vi "CheckForBadVIs.vi"() -> ()   [LabVIEW 2020]
panel:
  out "Bad":path[](array[path])=[path "ClassProviders/DesignPatterns/ActiveObjects/ActiveObjects_DynamicEvents_SubVIs/ActiveObjects_DynamicEvents_ControlWindow_4x4x4.vi", path "ClassProviders/DesignPatterns/ActiveObjects/ActiveObjects_DynamicEvents_SubVIs/ActiveObjects_DynamicEvents_ControlWindow_4x4x4_Singleton.vi", path "ClassProviders/DesignPatterns/ActiveObjects/ActiveObjects_DynamicEvents_SubVIs/ActiveObjects_DynamicEvents_ControlWindow_6x8x6.vi", path "ClassProviders/DesignPatterns/ActiveObjects/ActiveObjects_DynamicEvents_SubVIs/ActiveObjects_DynamicEvents_ControlWindow_6x8x6_Singleton.vi", path "ClassProviders/DesignPatterns/ActiveObjects/ActiveObjects_DynamicEvents_SubVIs/ActiveObjects_DynamicEvents_Process.vi", path "ClassProviders/DesignPatterns/ActiveObjects/ActiveObjects_DynamicEvents_SubVIs/ActiveObjects_DynamicEvents_ProcessRepository_EndevoGoop3.vi", path "ClassProviders/DesignPatterns/ActiveObjects/ActiveObjects_DynamicEvents_SubVIs/ActiveObjects_DynamicEvents_ProcessRepository_Native.vi", path "ClassProviders/DesignPatterns/ActiveObjects/ActiveObjects_DynamicEvents_SubVIs/ActiveObjects_DynamicEvents_SendMsgToProcess_4x4x4.vi", path "ClassProviders/DesignPatterns/ActiveObjects/ActiveObjects_DynamicEvents_SubVIs/ActiveObjects_DynamicEvents_SendMsgToProcess_4x4x4_Singleton.vi", path "ClassProviders/DesignPatterns/ActiveObjects/ActiveObjects_DynamicEvents_SubVIs/ActiveObjects_DynamicEvents_SendMsgToProcess_6x8x6.vi", path "ClassProviders/DesignPatterns/ActiveObjects/ActiveObjects_DynamicEvents_SubVIs/ActiveObjects_DynamicEvents_SendMsgToProcess_6x8x6_Singleton.vi", path "ClassProviders/DesignPatterns/ActiveObjects/ActiveObjects_DynamicEvents_SubVIs/ActiveObjects_DynamicEvents_StartProcess_OnePerClass.vi", path "ClassProviders/DesignPatterns/ActiveObjects/ActiveObjects_DynamicEvents_SubVIs/ActiveObjects_DynamicEvents_StartProcess_OnePerObject.vi", path "ClassProviders/DesignPatterns/ActiveObjects/ActiveObjects_DynamicEvents_SubVIs/ActiveObjects_DynamicEvents_StopProcess.vi", path "ClassProviders/DesignPatterns/ActiveObjects/ActiveObjects_Finisar_SubVIs/ActiveObjects_Finisar_ControlWindow_4x4x4.vi", path "ClassProviders/DesignPatterns/ActiveObjects/ActiveObjects_Finisar_SubVIs/ActiveObjects_Finisar_ControlWindow_4x4x4_Singleton.vi", path "ClassProviders/DesignPatterns/ActiveObjects/ActiveObjects_Finisar_SubVIs/ActiveObjects_Finisar_ControlWindow_6x8x6.vi", path "ClassProviders/DesignPatterns/ActiveObjects/ActiveObjects_Finisar_SubVIs/ActiveObjects_Finisar_ControlWindow_6x8x6_Singleton.vi", path "ClassProviders/DesignPatterns/ActiveObjects/ActiveObjects_Finisar_SubVIs/ActiveObjects_Finisar_Process.vi", path "ClassProviders/DesignPatterns/ActiveObjects/ActiveObjects_Finisar_SubVIs/ActiveObjects_Finisar_ProcessRepository_EndevoGoop3.vi", path "ClassProviders/DesignPatterns/ActiveObjects/ActiveObjects_Finisar_SubVIs/ActiveObjects_Finisar_ProcessRepository_Native.vi", path "ClassProviders/DesignPatterns/ActiveObjects/ActiveObjects_Finisar_SubVIs/ActiveObjects_Finisar_SendMsgToProcess2_4x4x4.vi", path "ClassProviders/DesignPatterns/ActiveObjects/ActiveObjects_Finisar_SubVIs/ActiveObjects_Finisar_SendMsgToProcess2_4x4x4_Singleton.vi", path "ClassProviders/DesignPatterns/ActiveObjects/ActiveObjects_Finisar_SubVIs/ActiveObjects_Finisar_SendMsgToProcess2_6x8x6.vi", path "ClassProviders/DesignPatterns/ActiveObjects/ActiveObjects_Finisar_SubVIs/ActiveObjects_Finisar_SendMsgToProcess2_6x8x6_Singleton.vi", path "ClassProviders/DesignPatterns/ActiveObjects/ActiveObjects_Finisar_SubVIs/ActiveObjects_Finisar_SendMsgToProcess_4x4x4.vi", path "ClassProviders/DesignPatterns/ActiveObjects/ActiveObjects_Finisar_SubVIs/ActiveObjects_Finisar_SendMsgToProcess_4x4x4_Singleton.vi", path "ClassProviders/DesignPatterns/ActiveObjects/ActiveObjects_Finisar_SubVIs/ActiveObjects_Finisar_SendMsgToProcess_6x8x6.vi", path "ClassProviders/DesignPatterns/ActiveObjects/ActiveObjects_Finisar_SubVIs/ActiveObjects_Finisar_SendMsgToProcess_6x8x6_Singleton.vi", path "ClassProviders/DesignPatterns/ActiveObjects/ActiveObjects_Finisar_SubVIs/ActiveObjects_Finisar_StartProcess_OnePerClass.vi", path "ClassProviders/DesignPatterns/ActiveObjects/ActiveObjects_Finisar_SubVIs/ActiveObjects_Finisar_StartProcess_OnePerObject.vi", path "ClassProviders/DesignPatterns/ActiveObjects/ActiveObjects_Finisar_SubVIs/ActiveObjects_Finisar_StopProcess.vi", path "ClassProviders/DesignPatterns/ActiveObjects/ActiveObjects_QueueQueue_SubVIs/ActiveObject_QueueQueue_Process.vi", path "ClassProviders/DesignPatterns/ActiveObjects/ActiveObjects_QueueQueue_SubVIs/ActiveObject_QueueQueue_ProcessRepository_EndevoGoop3.vi", path "ClassProviders/DesignPatterns/ActiveObjects/ActiveObjects_QueueQueue_SubVIs/ActiveObject_QueueQueue_ProcessRepository_Native.vi", path "ClassProviders/DesignPatterns/ActiveObjects/ActiveObjects_QueueQueue_SubVIs/ActiveObject_QueueQueue_ProcessRepository_OGoop.vi", path "ClassProviders/DesignPatterns/ActiveObjects/ActiveObjects_QueueQueue_SubVIs/ActiveObject_QueueQueue_StartProcess_OnePerClass.vi", path "ClassProviders/DesignPatterns/ActiveObjects/ActiveObjects_QueueQueue_SubVIs/ActiveObject_QueueQueue_StartProcess_OnePerObject.vi", path "ClassProviders/DesignPatterns/ActiveObjects/ActiveObjects_QueueQueue_SubVIs/ActiveObject_QueueQueue_StopProcess.vi", path "ClassProviders/DesignPatterns/ActiveObjects/ActiveObjects_QueueQueue_SubVIs/ActiveObjects_QueueQueue_SendMsgToProcess_4x4x4.vi", path "ClassProviders/DesignPatterns/ActiveObjects/ActiveObjects_QueueQueue_SubVIs/ActiveObjects_QueueQueue_SendMsgToProcess_4x4x4_Singleton.vi", path "ClassProviders/DesignPatterns/ActiveObjects/ActiveObjects_QueueQueue_SubVIs/ActiveObjects_QueueQueue_SendMsgToProcess_6x8x6.vi", path "ClassProviders/DesignPatterns/ActiveObjects/ActiveObjects_QueueQueue_SubVIs/ActiveObjects_QueueQueue_SendMsgToProcess_6x8x6_Singleton.vi", path "ClassProviders/DesignPatterns/GOOPDebugger/GOOPDebugger_SubVIs/GOOPDebugger_GetObjectStatus_4x4x4.vi", path "ClassProviders/DesignPatterns/GOOPDebugger/GOOPDebugger_SubVIs/GOOPDebugger_GetObjectStatus_6x8x6.vi", path "ClassProviders/DesignPatterns/Interface/Interface_SubVIs/Interface_GetReference_4x4x4.vi", path "ClassProviders/DesignPatterns/Interface/Interface_SubVIs/Interface_GetReference_6x8x6.vi", path "ClassProviders/DesignPatterns/Interface/Interface_SubVIs/Interface_Implement.vi", path "ClassProviders/DesignPatterns/Persistent/Persistent_SubVIs/Persistent_CreateReference_4x4x4.vi", path "ClassProviders/DesignPatterns/Persistent/Persistent_SubVIs/Persistent_CreateReference_6x8x6.vi", path "ClassProviders/DesignPatterns/Persistent/Persistent_SubVIs/Persistent_New_4x4x4.vi", path "ClassProviders/DesignPatterns/Persistent/Persistent_SubVIs/Persistent_New_6x8x6.vi", path "ClassProviders/DesignPatterns/ReferencedVariables/ReferencedVariables_SubVIs/ReferencedVariables_CreateReferenceVariable_4x4x4.vi", path "ClassProviders/DesignPatterns/ReferencedVariables/ReferencedVariables_SubVIs/ReferencedVariables_CreateReferenceVariable_6x8x6.vi", path "ClassProviders/DesignPatterns/ReferencedVariables/ReferencedVariables_SubVIs/ReferencedVariables_DeleteReferenceVariable_4x4x4.vi", path "ClassProviders/DesignPatterns/ReferencedVariables/ReferencedVariables_SubVIs/ReferencedVariables_DeleteReferenceVariable_6x8x6.vi", path "ClassProviders/DesignPatterns/ReferencedVariables/ReferencedVariables_SubVIs/ReferencedVariables_ReadReferencedVariable_4x4x4.vi", path "ClassProviders/DesignPatterns/ReferencedVariables/ReferencedVariables_SubVIs/ReferencedVariables_ReadReferencedVariable_4x4x4_Singleton.vi", path "ClassProviders/DesignPatterns/ReferencedVariables/ReferencedVariables_SubVIs/ReferencedVariables_ReadReferencedVariable_6x8x6.vi", path "ClassProviders/DesignPatterns/ReferencedVariables/ReferencedVariables_SubVIs/ReferencedVariables_ReadReferencedVariable_6x8x6_Singleton.vi", path "ClassProviders/DesignPatterns/ReferencedVariables/ReferencedVariables_SubVIs/ReferencedVariables_ReadWriteReferencedVariable_4x4x4.vi", path "ClassProviders/DesignPatterns/ReferencedVariables/ReferencedVariables_SubVIs/ReferencedVariables_ReadWriteReferencedVariable_4x4x4_Singleton.vi", path "ClassProviders/DesignPatterns/ReferencedVariables/ReferencedVariables_SubVIs/ReferencedVariables_ReadWriteReferencedVariable_6x8x6.vi", path "ClassProviders/DesignPatterns/ReferencedVariables/ReferencedVariables_SubVIs/ReferencedVariables_ReadWriteReferencedVariable_6x8x6_Singleton.vi", path "ClassProviders/Provider_EndevoGOOP300/Templates/BaseTemplate/methods/B_GetProperty.vi", path "ClassProviders/Provider_EndevoGOOP300/Templates/BaseTemplate/methods/B_NoneModifing.vi", path "ClassProviders/Provider_EndevoGOOP300/Templates/BaseTemplate/methods/B_ReadAttribute.vi", path "ClassProviders/Provider_EndevoGOOP300/Templates/BaseTemplate/methods/B_ReadClassAttribute.vi", path "ClassProviders/Provider_EndevoGOOP300/Templates/BaseTemplate/methods/B_ReadProperty.vi", path "ClassProviders/Provider_EndevoGOOP300/Templates/BaseTemplate/methods/B_ReadWriteAttribute.vi", path "ClassProviders/Provider_EndevoGOOP300/Templates/BaseTemplate/methods/B_ReadWriteClassAttribute.vi", path "ClassProviders/Provider_EndevoGOOP300/Templates/BaseTemplate/methods/B_SetProperty.vi", path "ClassProviders/Provider_EndevoGOOP300/Templates/BaseTemplate/methods/B_WriteAttribute.vi", path "ClassProviders/Provider_EndevoGOOP300/Templates/BaseTemplate/methods/B_WriteClassAttribute.vi", path "ClassProviders/Provider_EndevoGOOP300/Templates/BaseTemplate/methods/B_WriteProperty.vi", path "ClassProviders/Provider_EndevoGOOP300/Templates/BaseTemplate_4x4x4/methods/B_GetProperty.vi", path "ClassProviders/Provider_EndevoGOOP300/Templates/BaseTemplate_4x4x4/methods/B_NoneModifing.vi", path "ClassProviders/Provider_EndevoGOOP300/Templates/BaseTemplate_4x4x4/methods/B_ReadAttribute.vi", path "ClassProviders/Provider_EndevoGOOP300/Templates/BaseTemplate_4x4x4/methods/B_ReadClassAttribute.vi", path "ClassProviders/Provider_EndevoGOOP300/Templates/BaseTemplate_4x4x4/methods/B_ReadProperty.vi", path "ClassProviders/Provider_EndevoGOOP300/Templates/BaseTemplate_4x4x4/methods/B_ReadWriteAttribute.vi", path "ClassProviders/Provider_EndevoGOOP300/Templates/BaseTemplate_4x4x4/methods/B_ReadWriteClassAttribute.vi", path "ClassProviders/Provider_EndevoGOOP300/Templates/BaseTemplate_4x4x4/methods/B_SetProperty.vi", path "ClassProviders/Provider_EndevoGOOP300/Templates/BaseTemplate_4x4x4/methods/B_WriteAttribute.vi", path "ClassProviders/Provider_EndevoGOOP300/Templates/BaseTemplate_4x4x4/methods/B_WriteClassAttribute.vi", path "ClassProviders/Provider_EndevoGOOP300/Templates/BaseTemplate_4x4x4/methods/B_WriteProperty.vi", path "ClassProviders/Provider_EndevoGOOP300/Templates/SingletonTemplate/methods/Sgl_GetProperty.vi", path "ClassProviders/Provider_EndevoGOOP300/Templates/SingletonTemplate/methods/Sgl_NoneModifing.vi", path "ClassProviders/Provider_EndevoGOOP300/Templates/SingletonTemplate/methods/Sgl_ReadAttribute.vi", path "ClassProviders/Provider_EndevoGOOP300/Templates/SingletonTemplate/methods/Sgl_ReadWriteAttribute.vi", path "ClassProviders/Provider_EndevoGOOP300/Templates/SingletonTemplate/methods/Sgl_SetProperty.vi", path "ClassProviders/Provider_EndevoGOOP300/Templates/SingletonTemplate/methods/Sgl_WriteAttribute.vi", path "ClassProviders/Provider_EndevoGOOP300/Templates/SubTemplate/methods/S_GetProperty.vi", path "ClassProviders/Provider_EndevoGOOP300/Templates/SubTemplate/methods/S_NoneModifing.vi", path "ClassProviders/Provider_EndevoGOOP300/Templates/SubTemplate/methods/S_ReadAttribute.vi", path "ClassProviders/Provider_EndevoGOOP300/Templates/SubTemplate/methods/S_ReadClassAttribute.vi", path "ClassProviders/Provider_EndevoGOOP300/Templates/SubTemplate/methods/S_ReadProperty.vi", path "ClassProviders/Provider_EndevoGOOP300/Templates/SubTemplate/methods/S_ReadWriteAttribute.vi", path "ClassProviders/Provider_EndevoGOOP300/Templates/SubTemplate/methods/S_ReadWriteClassAttribute.vi", path "ClassProviders/Provider_EndevoGOOP300/Templates/SubTemplate/methods/S_SetProperty.vi", path "ClassProviders/Provider_EndevoGOOP300/Templates/SubTemplate/methods/S_WriteAttribute.vi", path "ClassProviders/Provider_EndevoGOOP300/Templates/SubTemplate/methods/S_WriteClassAttribute.vi", path "ClassProviders/Provider_EndevoGOOP300/Templates/SubTemplate/methods/S_WriteProperty.vi", path "ClassProviders/Provider_EndevoGOOP300/Templates/SubTemplate_4x4x4/methods/S_GetProperty.vi", path "ClassProviders/Provider_EndevoGOOP300/Templates/SubTemplate_4x4x4/methods/S_NoneModifing.vi", path "ClassProviders/Provider_EndevoGOOP300/Templates/SubTemplate_4x4x4/methods/S_ReadAttribute.vi", path "ClassProviders/Provider_EndevoGOOP300/Templates/SubTemplate_4x4x4/methods/S_ReadClassAttribute.vi", path "ClassProviders/Provider_EndevoGOOP300/Templates/SubTemplate_4x4x4/methods/S_ReadProperty.vi", path "ClassProviders/Provider_EndevoGOOP300/Templates/SubTemplate_4x4x4/methods/S_ReadWriteAttribute.vi", path "ClassProviders/Provider_EndevoGOOP300/Templates/SubTemplate_4x4x4/methods/S_ReadWriteClassAttribute.vi", path "ClassProviders/Provider_EndevoGOOP300/Templates/SubTemplate_4x4x4/methods/S_SetProperty.vi", path "ClassProviders/Provider_EndevoGOOP300/Templates/SubTemplate_4x4x4/methods/S_WriteAttribute.vi", path "ClassProviders/Provider_EndevoGOOP300/Templates/SubTemplate_4x4x4/methods/S_WriteClassAttribute.vi", path "ClassProviders/Provider_EndevoGOOP300/Templates/SubTemplate_4x4x4/methods/S_WriteProperty.vi", path "ClassProviders/Provider_EndevoGOOP400/Templates/G4BaseTemplate_Simple_4x4x4/methods/G4BaseTemplate_Simple_4x4x4_GetProperty.vi", path "ClassProviders/Provider_EndevoGOOP400/Templates/G4BaseTemplate_Simple_4x4x4/methods/G4BaseTemplate_Simple_4x4x4_NoneModifing.vi", path "ClassProviders/Provider_EndevoGOOP400/Templates/G4BaseTemplate_Simple_4x4x4/methods/G4BaseTemplate_Simple_4x4x4_ReadAttribute.vi", path "ClassProviders/Provider_EndevoGOOP400/Templates/G4BaseTemplate_Simple_4x4x4/methods/G4BaseTemplate_Simple_4x4x4_ReadProperty.vi", path "ClassProviders/Provider_EndevoGOOP400/Templates/G4BaseTemplate_Simple_4x4x4/methods/G4BaseTemplate_Simple_4x4x4_ReadWriteAttribute.vi", path "ClassProviders/Provider_EndevoGOOP400/Templates/G4BaseTemplate_Simple_4x4x4/methods/G4BaseTemplate_Simple_4x4x4_SetProperty.vi", path "ClassProviders/Provider_EndevoGOOP400/Templates/G4BaseTemplate_Simple_4x4x4/methods/G4BaseTemplate_Simple_4x4x4_WriteAttribute.vi", path "ClassProviders/Provider_EndevoGOOP400/Templates/G4BaseTemplate_Simple_4x4x4/methods/G4BaseTemplate_Simple_4x4x4_WriteProperty.vi", path "ClassProviders/Provider_EndevoGOOP400/Templates/G4BaseTemplate_Simple_6x8x6/methods/G4BaseTemplate_Simple_6x8x6_GetProperty.vi", path "ClassProviders/Provider_EndevoGOOP400/Templates/G4BaseTemplate_Simple_6x8x6/methods/G4BaseTemplate_Simple_6x8x6_NoneModifing.vi", path "ClassProviders/Provider_EndevoGOOP400/Templates/G4BaseTemplate_Simple_6x8x6/methods/G4BaseTemplate_Simple_6x8x6_ReadAttribute.vi", path "ClassProviders/Provider_EndevoGOOP400/Templates/G4BaseTemplate_Simple_6x8x6/methods/G4BaseTemplate_Simple_6x8x6_ReadProperty.vi", path "ClassProviders/Provider_EndevoGOOP400/Templates/G4BaseTemplate_Simple_6x8x6/methods/G4BaseTemplate_Simple_6x8x6_ReadWriteAttribute.vi", path "ClassProviders/Provider_EndevoGOOP400/Templates/G4BaseTemplate_Simple_6x8x6/methods/G4BaseTemplate_Simple_6x8x6_SetProperty.vi", path "ClassProviders/Provider_EndevoGOOP400/Templates/G4BaseTemplate_Simple_6x8x6/methods/G4BaseTemplate_Simple_6x8x6_WriteAttribute.vi", path "ClassProviders/Provider_EndevoGOOP400/Templates/G4BaseTemplate_Simple_6x8x6/methods/G4BaseTemplate_Simple_6x8x6_WriteProperty.vi", path "ClassProviders/Provider_EndevoGOOP400/Templates/G4BaseTemplate_Singleton_4x4x4/methods/G4BaseTemplate_Singleton_4x4x4_GetProperty.vi", path "ClassProviders/Provider_EndevoGOOP400/Templates/G4BaseTemplate_Singleton_4x4x4/methods/G4BaseTemplate_Singleton_4x4x4_ReadAttribute.vi", path "ClassProviders/Provider_EndevoGOOP400/Templates/G4BaseTemplate_Singleton_4x4x4/methods/G4BaseTemplate_Singleton_4x4x4_ReadWriteAttribute.vi", path "ClassProviders/Provider_EndevoGOOP400/Templates/G4BaseTemplate_Singleton_4x4x4/methods/G4BaseTemplate_Singleton_4x4x4_SetProperty.vi", path "ClassProviders/Provider_EndevoGOOP400/Templates/G4BaseTemplate_Singleton_4x4x4/methods/G4BaseTemplate_Singleton_4x4x4_WriteAttribute.vi", path "ClassProviders/Provider_EndevoGOOP400/Templates/G4BaseTemplate_Singleton_6x8x6/methods/G4BaseTemplate_Singleton_6x8x6_GetProperty.vi", path "ClassProviders/Provider_EndevoGOOP400/Templates/G4BaseTemplate_Singleton_6x8x6/methods/G4BaseTemplate_Singleton_6x8x6_ReadAttribute.vi", path "ClassProviders/Provider_EndevoGOOP400/Templates/G4BaseTemplate_Singleton_6x8x6/methods/G4BaseTemplate_Singleton_6x8x6_ReadWriteAttribute.vi", path "ClassProviders/Provider_EndevoGOOP400/Templates/G4BaseTemplate_Singleton_6x8x6/methods/G4BaseTemplate_Singleton_6x8x6_SetProperty.vi", path "ClassProviders/Provider_EndevoGOOP400/Templates/G4BaseTemplate_Singleton_6x8x6/methods/G4BaseTemplate_Singleton_6x8x6_WriteAttribute.vi", path "ClassProviders/Provider_EndevoGOOP400/Templates/G4InterfaceTemplate_4x4x4/methods/G4InterfaceTemplate_4x4x4_Method.vi", path "ClassProviders/Provider_EndevoGOOP400/Templates/G4InterfaceTemplate_6x8x6/methods/G4InterfaceTemplate_6x8x6_Method.vi", path "ClassProviders/Provider_EndevoGOOP400/Templates/G4SubTemplate_Simple_4x4x4/methods/G4SubTemplate_Simple_4x4x4_GetProperty.vi", path "ClassProviders/Provider_EndevoGOOP400/Templates/G4SubTemplate_Simple_4x4x4/methods/G4SubTemplate_Simple_4x4x4_NoneModifing.vi", path "ClassProviders/Provider_EndevoGOOP400/Templates/G4SubTemplate_Simple_4x4x4/methods/G4SubTemplate_Simple_4x4x4_ReadAttribute.vi", path "ClassProviders/Provider_EndevoGOOP400/Templates/G4SubTemplate_Simple_4x4x4/methods/G4SubTemplate_Simple_4x4x4_ReadProperty.vi", path "ClassProviders/Provider_EndevoGOOP400/Templates/G4SubTemplate_Simple_4x4x4/methods/G4SubTemplate_Simple_4x4x4_ReadWriteAttribute.vi", path "ClassProviders/Provider_EndevoGOOP400/Templates/G4SubTemplate_Simple_4x4x4/methods/G4SubTemplate_Simple_4x4x4_SetProperty.vi", path "ClassProviders/Provider_EndevoGOOP400/Templates/G4SubTemplate_Simple_4x4x4/methods/G4SubTemplate_Simple_4x4x4_WriteAttribute.vi", path "ClassProviders/Provider_EndevoGOOP400/Templates/G4SubTemplate_Simple_4x4x4/methods/G4SubTemplate_Simple_4x4x4_WriteProperty.vi", path "ClassProviders/Provider_EndevoGOOP400/Templates/G4SubTemplate_Simple_6x8x6/methods/G4SubTemplate_Simple_6x8x6_GetProperty.vi", path "ClassProviders/Provider_EndevoGOOP400/Templates/G4SubTemplate_Simple_6x8x6/methods/G4SubTemplate_Simple_6x8x6_NoneModifing.vi", path "ClassProviders/Provider_EndevoGOOP400/Templates/G4SubTemplate_Simple_6x8x6/methods/G4SubTemplate_Simple_6x8x6_ReadAttribute.vi", path "ClassProviders/Provider_EndevoGOOP400/Templates/G4SubTemplate_Simple_6x8x6/methods/G4SubTemplate_Simple_6x8x6_ReadProperty.vi", path "ClassProviders/Provider_EndevoGOOP400/Templates/G4SubTemplate_Simple_6x8x6/methods/G4SubTemplate_Simple_6x8x6_ReadWriteAttribute.vi", path "ClassProviders/Provider_EndevoGOOP400/Templates/G4SubTemplate_Simple_6x8x6/methods/G4SubTemplate_Simple_6x8x6_SetProperty.vi", path "ClassProviders/Provider_EndevoGOOP400/Templates/G4SubTemplate_Simple_6x8x6/methods/G4SubTemplate_Simple_6x8x6_WriteAttribute.vi", path "ClassProviders/Provider_EndevoGOOP400/Templates/G4SubTemplate_Simple_6x8x6/methods/G4SubTemplate_Simple_6x8x6_WriteProperty.vi", path "ClassProviders/Provider_EndevoGOOP400/Templates/G4SubTemplate_Singleton_4x4x4/methods/G4SubTemplate_Singleton_4x4x4_GetProperty.vi", path "ClassProviders/Provider_EndevoGOOP400/Templates/G4SubTemplate_Singleton_4x4x4/methods/G4SubTemplate_Singleton_4x4x4_ReadAttribute.vi", path "ClassProviders/Provider_EndevoGOOP400/Templates/G4SubTemplate_Singleton_4x4x4/methods/G4SubTemplate_Singleton_4x4x4_ReadWriteAttribute.vi", path "ClassProviders/Provider_EndevoGOOP400/Templates/G4SubTemplate_Singleton_4x4x4/methods/G4SubTemplate_Singleton_4x4x4_SetProperty.vi", path "ClassProviders/Provider_EndevoGOOP400/Templates/G4SubTemplate_Singleton_4x4x4/methods/G4SubTemplate_Singleton_4x4x4_WriteAttribute.vi", path "ClassProviders/Provider_EndevoGOOP400/Templates/G4SubTemplate_Singleton_6x8x6/methods/G4SubTemplate_Singleton_6x8x6_GetProperty.vi", path "ClassProviders/Provider_EndevoGOOP400/Templates/G4SubTemplate_Singleton_6x8x6/methods/G4SubTemplate_Singleton_6x8x6_ReadAttribute.vi", path "ClassProviders/Provider_EndevoGOOP400/Templates/G4SubTemplate_Singleton_6x8x6/methods/G4SubTemplate_Singleton_6x8x6_ReadWriteAttribute.vi", path "ClassProviders/Provider_EndevoGOOP400/Templates/G4SubTemplate_Singleton_6x8x6/methods/G4SubTemplate_Singleton_6x8x6_SetProperty.vi", path "ClassProviders/Provider_EndevoGOOP400/Templates/G4SubTemplate_Singleton_6x8x6/methods/G4SubTemplate_Singleton_6x8x6_WriteAttribute.vi", path "UML/AbstractEdge_class/utils/AbstractEdge_Delete.vi", path "UML/AbstractEdge_class/utils/AbstractEdge_GetAttributesToModify.vi", path "UML/AbstractEdge_class/utils/AbstractEdge_GetClassAttributes.vi", path "UML/AbstractEdge_class/utils/AbstractEdge_GetClassAttributesToModify.vi", path "UML/AbstractEdge_class/utils/AbstractEdge_GOOPKernel.vi", path "UML/AbstractEdge_class/utils/AbstractEdge_SetModifiedAttributes.vi", path "UML/AbstractEdge_class/utils/AbstractEdge_SetModifiedClassAttributes.vi", path "UML/CallEdge_class/utils/CallEdge_CastToMoreSpecific.vi", path "UML/CallEdge_class/utils/CallEdge_CreateReference.vi", path "UML/CallEdge_class/utils/CallEdge_Delete.vi", path "UML/CallEdge_class/utils/CallEdge_GetAttributesToModify.vi", path "UML/CallEdge_class/utils/CallEdge_GetClassAttributes.vi", path "UML/CallEdge_class/utils/CallEdge_GetClassAttributesToModify.vi", path "UML/CallEdge_class/utils/CallEdge_GOOPKernel.vi", path "UML/CallEdge_class/utils/CallEdge_SetModifiedAttributes.vi", path "UML/CallEdge_class/utils/CallEdge_SetModifiedClassAttributes.vi", path "UML/ClassRelationshipEdge_class/utils/ClassRelationshipEdge_CastToMoreSpecific.vi", path "UML/ClassRelationshipEdge_class/utils/ClassRelationshipEdge_CreateReference.vi", path "UML/ClassRelationshipEdge_class/utils/ClassRelationshipEdge_Delete.vi", path "UML/ClassRelationshipEdge_class/utils/ClassRelationshipEdge_GetAttributesToModify.vi", path "UML/ClassRelationshipEdge_class/utils/ClassRelationshipEdge_GetClassAttributes.vi", path "UML/ClassRelationshipEdge_class/utils/ClassRelationshipEdge_GetClassAttributesToModify.vi", path "UML/ClassRelationshipEdge_class/utils/ClassRelationshipEdge_GOOPKernel.vi", path "UML/ClassRelationshipEdge_class/utils/ClassRelationshipEdge_SetModifiedAttributes.vi", path "UML/ClassRelationshipEdge_class/utils/ClassRelationshipEdge_SetModifiedClassAttributes.vi", path "UML/GeneralPathEdge_class/utils/GeneralPathEdge_CastToMoreSpecific.vi", path "UML/GeneralPathEdge_class/utils/GeneralPathEdge_CreateReference.vi", path "UML/GeneralPathEdge_class/utils/GeneralPathEdge_Delete.vi", path "UML/GeneralPathEdge_class/utils/GeneralPathEdge_GetAttributesToModify.vi", path "UML/GeneralPathEdge_class/utils/GeneralPathEdge_GetClassAttributes.vi", path "UML/GeneralPathEdge_class/utils/GeneralPathEdge_GetClassAttributesToModify.vi", path "UML/GeneralPathEdge_class/utils/GeneralPathEdge_GOOPKernel.vi", path "UML/GeneralPathEdge_class/utils/GeneralPathEdge_SetModifiedAttributes.vi", path "UML/GeneralPathEdge_class/utils/GeneralPathEdge_SetModifiedClassAttributes.vi", path "UML/Graphics_class/utils/Graphics_Delete.vi", path "UML/Graphics_class/utils/Graphics_GetAttributesToModify.vi", path "UML/Graphics_class/utils/Graphics_GetClassAttributes.vi", path "UML/Graphics_class/utils/Graphics_GetClassAttributesToModify.vi", path "UML/Graphics_class/utils/Graphics_GetObjectStatus.vi", path "UML/Graphics_class/utils/Graphics_GOOPKernel.vi", path "UML/Graphics_class/utils/Graphics_SetModifiedAttributes.vi", path "UML/Graphics_class/utils/Graphics_SetModifiedClassAttributes.vi", path "UML/NoteEdge_class/utils/NoteEdge_CastToMoreSpecific.vi", path "UML/NoteEdge_class/utils/NoteEdge_Delete.vi", path "UML/NoteEdge_class/utils/NoteEdge_GetAttributesToModify.vi", path "UML/NoteEdge_class/utils/NoteEdge_GetClassAttributes.vi", path "UML/NoteEdge_class/utils/NoteEdge_GetClassAttributesToModify.vi", path "UML/NoteEdge_class/utils/NoteEdge_GetObjectStatus.vi", path "UML/NoteEdge_class/utils/NoteEdge_GOOPKernel.vi", path "UML/NoteEdge_class/utils/NoteEdge_SetModifiedAttributes.vi", path "UML/NoteEdge_class/utils/NoteEdge_SetModifiedClassAttributes.vi", path "UML/SegmentedLineEdge_class/utils/SegmentedLineEdge_CastToMoreSpecific.vi", path "UML/SegmentedLineEdge_class/utils/SegmentedLineEdge_CreateReference.vi", path "UML/SegmentedLineEdge_class/utils/SegmentedLineEdge_Delete.vi", path "UML/SegmentedLineEdge_class/utils/SegmentedLineEdge_GetAttributesToModify.vi", path "UML/SegmentedLineEdge_class/utils/SegmentedLineEdge_GetClassAttributes.vi", path "UML/SegmentedLineEdge_class/utils/SegmentedLineEdge_GetClassAttributesToModify.vi", path "UML/SegmentedLineEdge_class/utils/SegmentedLineEdge_GOOPKernel.vi", path "UML/SegmentedLineEdge_class/utils/SegmentedLineEdge_SetModifiedAttributes.vi", path "UML/SegmentedLineEdge_class/utils/SegmentedLineEdge_SetModifiedClassAttributes.vi", path "UML/StateTransitionEdge_class/utils/StateTransitionEdge_CastToMoreSpecific.vi", path "UML/StateTransitionEdge_class/utils/StateTransitionEdge_CreateReference.vi", path "UML/StateTransitionEdge_class/utils/StateTransitionEdge_Delete.vi", path "UML/StateTransitionEdge_class/utils/StateTransitionEdge_GetAttributesToModify.vi", path "UML/StateTransitionEdge_class/utils/StateTransitionEdge_GetClassAttributes.vi", path "UML/StateTransitionEdge_class/utils/StateTransitionEdge_GetClassAttributesToModify.vi", path "UML/StateTransitionEdge_class/utils/StateTransitionEdge_GOOPKernel.vi", path "UML/StateTransitionEdge_class/utils/StateTransitionEdge_SetModifiedAttributes.vi", path "UML/StateTransitionEdge_class/utils/StateTransitionEdge_SetModifiedClassAttributes.vi"]
  out "Modified":path[](array[path])
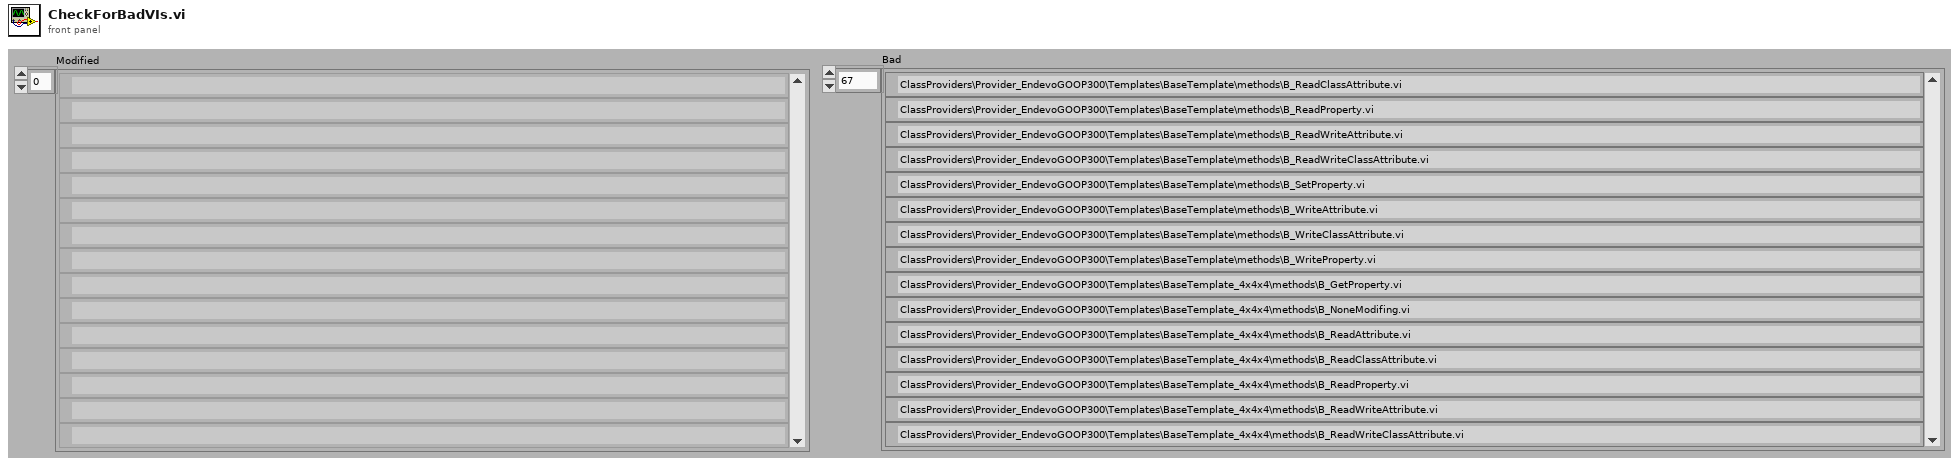
[diagram p1: front panel]
types:
  T1 = enum32{"Bad", "Idle", "Run top level", "Running"}
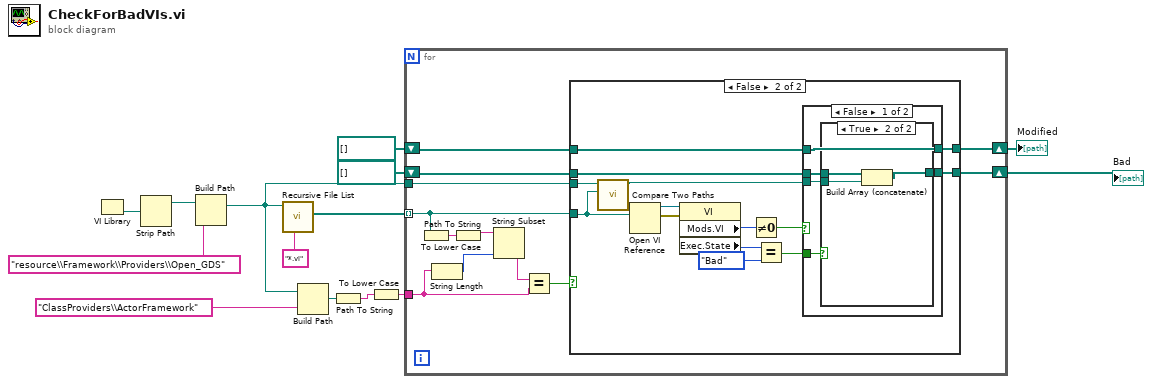
[diagram p0: block diagram]
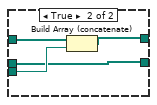
[diagram p4: hidden frame]
diagram:
  n1 = VI Library() -> (path=w14:path)
  n2 = Strip Path(path=w14) -> (stripped path=w13:path)  [unwired: 1 out]
  n3 = Build Path(base path=w13, name or relative path="resource\\Framework\\Providers\\Open_GDS") -> (appended path=w1:path)
  n4 = call <vilib>:"Recursive File List.vi"("pattern"="*.vi", "Folder Path"=w1) -> ("All Files in Dir"=w11:path[])  [unwired: 5 in, 4 out]
  n5 = Build Path(base path=w1, name or relative path="ClassProviders\\ActorFramework") -> (appended path=w8:path)
  n6 = Path To String(path=w8) -> (string=w9:string)
  n7 = To Lower Case(string=w9) -> (all lower case string=w7:string)
  n8 = for {
    tunnel: w11 -> [w26] mode=indexing
    tunnel: w7 -> [w16]
    shift-right: [w24] -> w3
    shift-left: path[] [] -> [w25]
    shift-right: [w23] -> w4
    shift-left: path[] [] -> [w22]
    tunnel: w1 -> [w21]
    n9 = Path To String(path=w26) -> (string=w20:string)
    n10 = String Length(string=w16) -> (length=w18:i32)
    n11 = To Lower Case(string=w20) -> (all lower case string=w19:string)
    n12 = String Subset(string=w19, length (rest)=w18) -> (substring=w17:string)  [unwired: 1 in]
    n13 = Equal?(x=w17, y=w16) -> (x = y?=w15:bool)
    n14 = case shown="False" w15 {
      tunnel: w26 -> [_ w30]
      tunnel: w25 -> [w28 w35]
      tunnel: [w28 w34] -> w24
      tunnel: w22 -> [w27 w32]
      tunnel: [w27 w33] -> w23
      tunnel: w21 -> [_ w31]
      frame True {
      }
      frame False {
        n15 = call <vilib>:"Compare Two Paths.vi"("Path 2"=w30, "Path 1"=w31) -> ("Relative Path from 1 to 2"=w29:path)  [unwired: 6 in, 3 out]
        n16 = Open VI Reference(vi path=w30) -> (vi reference=w42:refnum<vi>, error out=w41:errorcluster)  [unwired: 5 in]
        n17 = property class="VI"(reference=w42, error in=w41) -> ("Mods.VI"=w40:u64, "Exec.State"=w39:T1)  [unwired: 2 out]
        n18 = Not Equal To 0?(x=w40) -> (x != 0?=w37:bool)
        n19 = Equal?(x=w39, y=T1."Bad") -> (x = y?=w36:bool)
        n20 = case shown="False" w37 {
          tunnel: w36 -> [w47 _]
          tunnel: w29 -> [w46 w53]
          tunnel: w35 -> [w45 w52]
          tunnel: [w44 w52] -> w34
          tunnel: w32 -> [w43 w55]
          tunnel: [w43 w54] -> w33
          frame False {
            n21 = case shown="True" w47 {
              tunnel: w46 -> [_ w51]
              tunnel: w45 -> [w48 w50]
              tunnel: [w48 w49] -> w44
              frame False {
              }
              frame True {
                n22 = Build Array (concatenate)(w50, w51) -> (w49:path[])
              }
            }
          }
          frame True {
            n23 = Build Array (concatenate)(w55, w53) -> (w54:path[])
          }
        }
      }
    }
  }
  "Modified" <- w4
  "Bad" <- w3
